vi "Add Channel to All Groups.vi"(7 "GUID (Default Channel)":string="03D3BB99-1485-13A6-561D1F898F032919", 8 "error in (no error)":errorcluster, 9 "Channel":T1, 10 "Channel Name":string, 11 "Item Ref in":T3 format="%.0x") -> (0 "error out":errorcluster, 3 "Item Ref out":T3 format="%.0x")   [LabVIEW 2017, in "DSF System Explorer.lvlib"]
uses:
  DSF System Explorer.lvlib
  <vilib>/NI Veristand/Custom Device API/Custom Device Item Ref.ctl
  <vilib>/NI Veristand/Custom Device API/Custom Device Channel.ctl
  <vilib>/NI Veristand/Custom Device API/Custom Device Channel Type.ctl
  <vilib>/NI Veristand/Custom Device API/Custom Device API.lvlib
  Shared/DSF Shared.lvlib
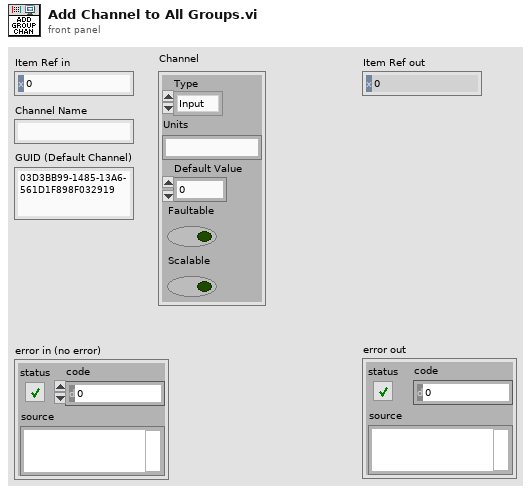
[diagram p1: front panel]
types:
  T1 = typedef "Custom Device API.lvlib/Custom Device Channel.ctl" = cluster{"Type":T2, "Units":string, "Default Value":dbl, "Faultable":bool, "Scalable":bool}
  T2 = typedef "Custom Device API.lvlib/Custom Device Channel Type.ctl" = enum16{"Input", "Output"}
  T3 = typedef "Custom Device API.lvlib/Custom Device Item Ref.ctl" = u64
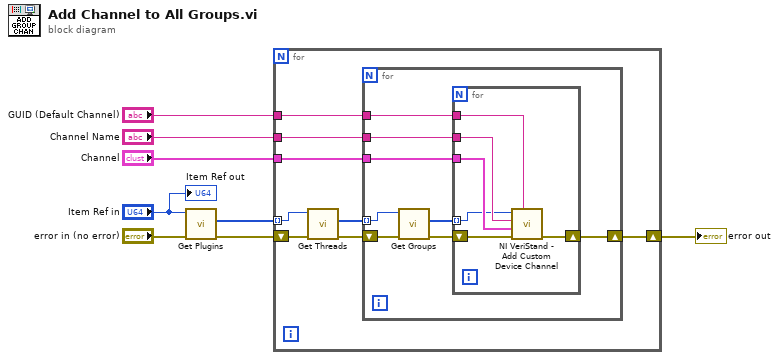
[diagram p0: block diagram]
diagram:
  n1 = call "Get Plugins.vi"("error in (no error)"="error in (no error)", "Item Ref in"="Item Ref in") -> ("error out"=w6:errorcluster, "Plugin refs"=w5:T3[])  [unwired: 7 in, 1 out]
  n2 = for {
    tunnel: w5 -> [w11] mode=indexing
    tunnel: "Channel Name" -> [w15]
    tunnel: "Channel" -> [w14]
    tunnel: "GUID (Default Channel)" -> [w13]
    shift-right: [w16] -> w4
    shift-left: w6 -> [w12]
    n3 = call "Get Threads.vi"("error in (no error)"=w12, "Item Ref in"=w11) -> ("error out"=w10:errorcluster, "Plugin refs"=w9:T3[])  [unwired: 7 in, 1 out]
    n4 = for {
      shift-right: [w21] -> w16
      shift-left: w10 -> [w24]
      tunnel: w9 -> [w23] mode=indexing
      tunnel: w15 -> [w20]
      tunnel: w14 -> [w19]
      tunnel: w13 -> [w18]
      n5 = call "Get Groups.vi"("error in (no error)"=w24, "Plugin Ref in"=w23) -> ("error out"=w22:errorcluster, "Group refs"=w17:T3[])  [unwired: 7 in, 1 out]
      n6 = for {
        shift-right: [w29] -> w21
        shift-left: w22 -> [w30]
        tunnel: w17 -> [w26] mode=indexing
        tunnel: w20 -> [w27]
        tunnel: w19 -> [w28]
        tunnel: w18 -> [w25]
        n7 = call <vilib>:"NI VeriStand - Add Custom Device Channel.vi"("GUID (Default Channel)"=w25, "error in (no error)"=w30, "Channel"=w28, "Channel Name"=w27, "Parent Ref in"=w26) -> ("error out"=w29:errorcluster)  [unwired: 3 in, 3 out]
      }
    }
  }
  "error out" <- w4
  "Item Ref out" <- "Item Ref in"
